vi "Read Marker (All Marker).vi"(0 "VISA resource name":refnum<visa-resource-name>, 11 "error in (no error)":errorcluster) -> (4 "VISA resource name out":refnum<visa-resource-name>, 6 "Marker Data Values":dbl[](array[numeric]) format="%.3f", 15 "error out":errorcluster)   [LabVIEW 2023, in "Anritsu Signal Analyzer Series.lvlib"]
doc: "Reads all Marker data."
uses:
  Anritsu Signal Analyzer Series.lvlib
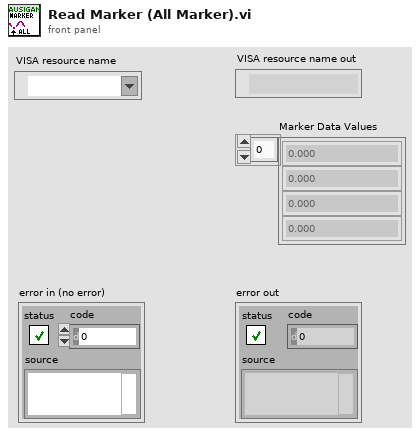
[diagram p1: front panel]
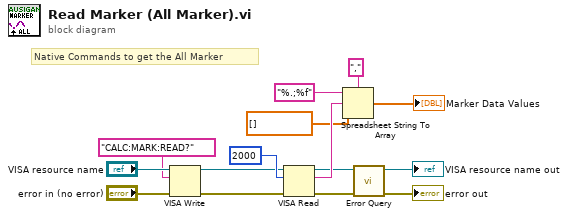
[diagram p0: block diagram]
diagram:
  # "Native Commands to get the All Marker"
  n1 = VISA Write(VISA resource name="VISA resource name", write buffer="CALC:MARK:READ?" ("_Command"), error in (no error)="error in (no error)") -> (VISA resource name out=w4:refnum<visa-resource-name>, error out=w5:errorcluster)  [unwired: 1 out]
  n2 = VISA Read(VISA resource name=w4, byte count=u32 2000 ("byte count (0)"), error in (no error)=w5) -> (VISA resource name out=w3:refnum<visa-resource-name>, read buffer=w10:string, error out=w2:errorcluster)  [unwired: 1 out]
  n3 = Spreadsheet String To Array(delimiter (Tab)=",", format string="%.;%f", spreadsheet string=w10, array type (2D Dbl)=dbl[] [] ("Values")) -> (array=→"Marker Data Values":dbl[])
  n4 = call "Error Query.vi"("error in (no error)"=w2, "VISA resource name"=w3) -> ("error out"=→"error out":errorcluster, "VISA resource name out"=→"VISA resource name out":refnum<visa-resource-name>)  [unwired: 6 in, 2 out]
